vi "Get Log Folder-old.vi"(8 "error in (no error)":errorcluster, 11 "Trace Controller in":refnum<class "Trace Controller.lvclass">) -> (0 "error out":errorcluster, 1 "Folder Found?":bool, 2 "Folder":path=path "C:/", 3 "Trace Controller out":refnum<class "Trace Controller.lvclass">)   [LabVIEW 2014, in "Robot Actor Framework.lvlib" / "Trace.lvlib" / "Trace Controller.lvclass"]
uses:
  Trace Controller.lvclass
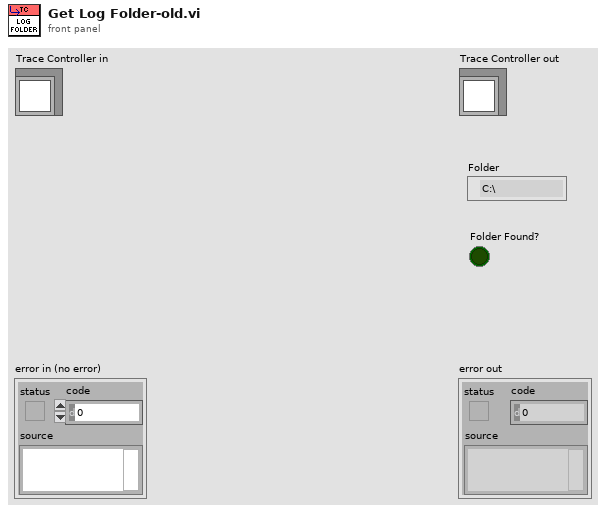
[diagram p1: front panel]
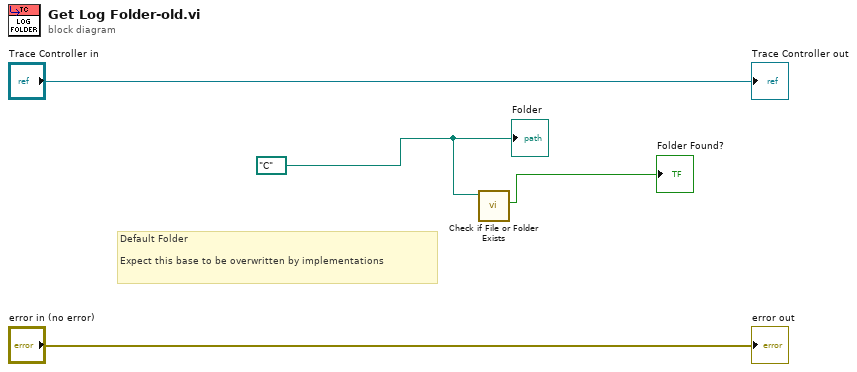
[diagram p0: block diagram]
diagram:
  w2 = path "C:/" ("Folder")
  # "Default Folder\n\nExpect this base to be overwritten by implementations"
  n1 = call <vilib>:"Check if File or Folder Exists.vi"("path"=w2) -> ("file or folder exists?"=→"Folder Found?":bool)  [unwired: 8 in, 2 out]
  "error out" <- "error in (no error)"
  "Trace Controller out" <- "Trace Controller in"
  "Folder" <- w2
